vi "ConfigDlg.vi"(8 "error in (no error)":errorcluster, 11 "FFT in":refnum<class "FFT.lvclass">) -> (0 "error out":errorcluster, 2 "Changed":bool, 3 "FFT out":refnum<class "FFT.lvclass">)   [LabVIEW 2018, in "AnalysisPlugins.lvlib" / "FFT.lvclass"]
uses:
  FFT.lvclass
  Y:/Projects/PMUCal/Modules/Analysis/AnalysisPlugins/AnalysisPluginBaseClass/AnalysisPluginsBase.lvclass
  C:/Program Files/National Instruments/LabVIEW 2018/user.lib/NIST/BaseClasses/BasePlugin_class/BasePlugin.lvclass
  FitterBaseClass/Typedefs/clAnalysisConfig.ctl
  Typedefs/FftView.ctl
  <vilib>/Analysis/4window.llb/windowTd.ctl
  AnalysisPluginBaseClass/AnalysisPluginsBase.lvclass/AnalysisPluginsBase.ctl
  FFT.lvclass/FFT.ctl
  <userlib>/NIST/BaseClasses/BasePlugin_class/BasePlugin.lvclass/BasePlugin.ctl
  AnalysisPluginBaseClass/Accessors/Read AnalysisConfig.vi
  Accessors/Read FftView.vi
  Accessors/Read WindowFunction.vi
  AnalysisPluginBaseClass/Accessors/Read Duration.vi
  <userlib>/NIST/BaseClasses/BasePlugin_class/Accessors/Read PluginIniFilePath.vi
  AnalysisPluginBaseClass/Accessors/Write AnalysisConfig.vi
  Accessors/Write FftView.vi
  Accessors/Write WindowFunction.vi
  AnalysisPluginBaseClass/Accessors/Write Duration.vi
  <vilib>/Utility/config.llb/NI_LVConfig.lvlib
  FitterBaseClass/FitterBase.lvclass
  <vilib>/Analysis/NI_AALPro.lvlib
panel:
  in  "Duration":dbl
  in  "WindowFunction":T1 items=["Rectangle"=0, "Hanning"=1, "Hamming"=2, "Blackman-Harris"=3, "Exact Blackman"=4, "Blackman"=5, "Flat Top"=6, "4 Term B-Harris "=7, "7 Term B-Harris"=8, "Low Sidelobe"=9, "Blackman Nuttall"=11, "Triangle"=30, "Bartlett-Hanning"=31, "Bohman"=32, "Parzen"=33, "Welch"=34, "Kaiser"=60, "Dolph-Chebyshev"=61, "Gaussian"=62]
  in  "FftView":T2
  in  "btnDone":bool
  in  "BtnCancel":bool
  in  "clAnalysisConfig":T3={"F0"=60, "SettlingTime"=7.0, "AnalysisCycles"=20.0, "SampleRate"=4800.0, "NumChannels"=6, "TsOffset"=enum."start"}
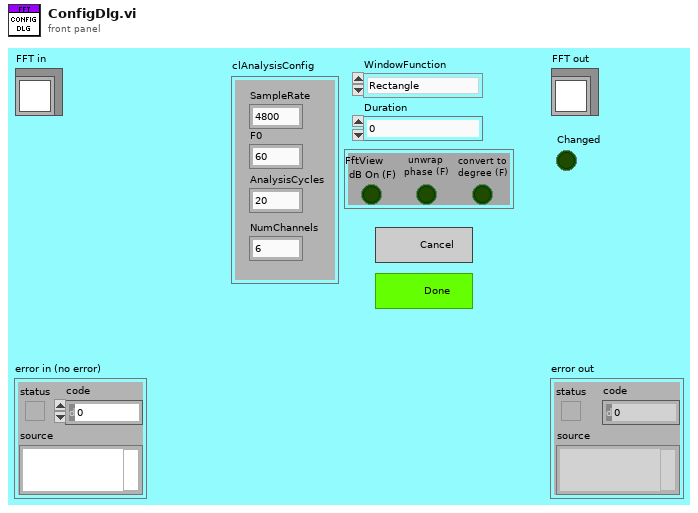
[diagram p1: front panel]
types:
  T1 = typedef "NI_AALPro.lvlib/windowTd.ctl" = u32
  T2 = typedef "AnalysisPlugins.lvlib/FFT.lvclass/FftView.ctl" = cluster{"dB On (F)":bool, "unwrap phase (F)":bool, "convert to degree (F)":bool}
  T3 = typedef "AnalysisPlugins.lvlib/FitterBase.lvclass/clAnalysisConfig.ctl" = cluster{"F0":u32, "SettlingTime":dbl, "AnalysisCycles":dbl, "SampleRate":dbl, "NumChannels":u32, "TsOffset":enum16{"start", "middle", "end"}}
  T4 = enum32{"Invalid", "Standard", "Closed", "Hidden", "Minimized", "Maximized"}
  T5 = enum32{"Invalid", "Default", "Floating", "Floating/Auto-Hide", "Modal"}
  T6 = typedef "NI_LVConfig.lvlib/Config Data RefNum.ctl" = refnum<k1>
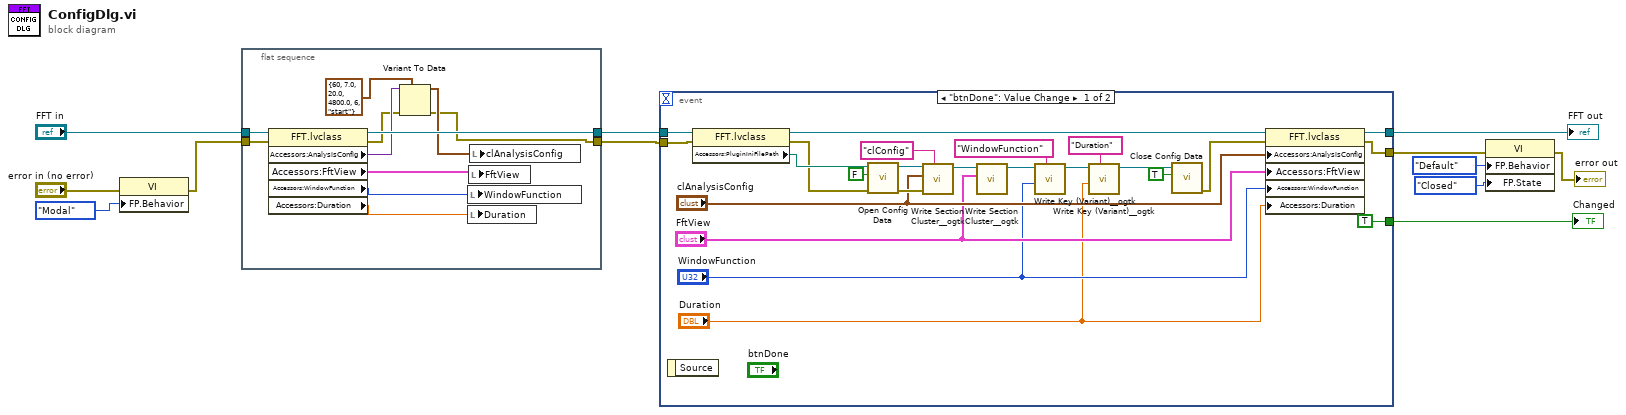
[diagram p0: block diagram]
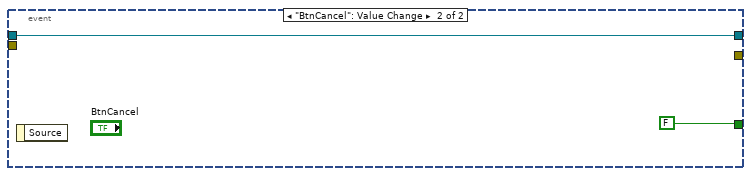
[diagram p2: hidden frame]
diagram:
  n1 = property class="VI"(error in="error in (no error)", "FP.Behavior"=T5."Modal" ("Front Panel Window:Behavior")) -> (error out=w10:errorcluster)  [unwired: 1 in, 1 out]
  n2 = flat-sequence {
    tunnel: w10 -> [w23]
    tunnel: "FFT in" -> [w22]
    tunnel: [w21] -> w8
    tunnel: [w14] -> w1
    frame #0 {
      n3 = property class="FFT.lvclass"(reference=w22, error in=w23) -> (reference out=w21:refnum<class "FFT.lvclass">, error out=w15:errorcluster, "Accessors:AnalysisConfig"=w17:variant, "Accessors:FftView"=w20:T2, "Accessors:WindowFunction"=w19:T1, "Accessors:Duration"=w18:dbl)
      n4 = Variant To Data(error in=w15, type=T3 {"F0"=60, "SettlingTime"=7.0, "AnalysisCycles"=20.0, "SampleRate"=4800.0, "NumChannels"=6, "TsOffset"=enum."start"} ("clAnalysisConfig"), Variant=w17) -> (data=w16:T3, error out=w14:errorcluster)
      n5 = local write "WindowFunction"(w19) -> ()
      n6 = local write "Duration"(w18) -> ()
      n7 = local write "FftView"(w20) -> ()
      n8 = local write "clAnalysisConfig"(w16) -> ()
    }
  }
  n9 = event shown="[0] \"btnDone\": Value Change" {
    selector: _ -> [_ _]
    dyn-events: _ -> [_ _]
    timeout: _ -> [_ _]
    tunnel: w8 -> [w47 w49]
    tunnel: [w36 w49] -> w6
    tunnel: [w35 _] -> w5
    tunnel: [TRUE FALSE] -> w7
    tunnel: w1 -> [w27 _]
    event "btnDone": Value Change {
      n10 = event-data() -> ()  [unwired: 1 in, 1 out]
      n11 = property class="FFT.lvclass"(reference=w47, error in=w27) -> (reference out=w39:refnum<class "FFT.lvclass">, error out=w40:errorcluster, "Accessors:PluginIniFilePath"=w41:path)
      n12 = call <vilib>:"Open Config Data.vi"("error in (no error)"=w40, "create file if necessary (T)"=FALSE, "configuration file path"=w41) -> ("error out"=w44:errorcluster, "refnum"=w45:T6)  [unwired: 6 in, 1 out]
      n13 = call <userlib>:"Write Section Cluster__ogtk.vi"("section (optional)"="clConfig", "error in (no error)"=w44, "Section Formatted Cluster"="clAnalysisConfig", "refnum"=w45) -> ("dup refnum"=w33:T6)  [unwired: 6 in, 1 out]
      n14 = call <userlib>:"Write Section Cluster__ogtk.vi"("Section Formatted Cluster"="FftView", "refnum"=w33) -> ("dup refnum"=w32:T6)  [unwired: 8 in, 1 out]
      n15 = call <userlib>:"Write Key (Variant)__ogtk.vi"("section"="WindowFunction", "key-value"="WindowFunction", "refnum"=w32) -> ("refnum out"=w31:T6)  [unwired: 7 in, 1 out]
      n16 = call <userlib>:"Write Key (Variant)__ogtk.vi"("section"="Duration", "key-value"="Duration", "refnum"=w31) -> ("refnum out"=w26:T6)  [unwired: 7 in, 1 out]
      n17 = call <vilib>:"Close Config Data.vi"("write file if changed (T)"=TRUE, "refnum"=w26) -> ("error out"=w37:errorcluster)  [unwired: 8 in, 1 out]
      n18 = property class="FFT.lvclass"(reference=w39, error in=w37, "Accessors:AnalysisConfig"="clAnalysisConfig", "Accessors:FftView"="FftView", "Accessors:WindowFunction"="WindowFunction", "Accessors:Duration"="Duration") -> (reference out=w36:refnum<class "FFT.lvclass">, error out=w35:errorcluster)
    }
    event "BtnCancel": Value Change {
      n19 = event-data() -> ()  [unwired: 1 in, 1 out]
    }
  }
  "FFT out" <- w6
  "Changed" <- w7
  n20 = property class="VI"(error in=w5, "FP.Behavior"=T5."Default" ("Front Panel Window:Behavior"), "FP.State"=T4."Closed" ("Front Panel Window:State")) -> (error out=→"error out":errorcluster)  [unwired: 1 in, 1 out]
